vi "Create.vi"(7 "options (all enabled)":T1={"Measure Period"=TRUE, "Measure Rx/Tx Duration"=TRUE}, 8 "error in (no error)":errorcluster) -> (0 "error out":errorcluster, 3 "performance":refnum<class "Performance.lvclass">)   [LabVIEW 2017, in "DSF Core.lvlib" / "Performance.lvclass"]
uses:
  Performance.lvclass
  Typedefs/DSF Performance Options.ctl
  Timing Status/Timing Status Data.ctl
  <vilib>/NI/Memory Manager/Classes/Pointer/Pointer.lvclass/Pointer.ctl
  Performance.lvclass/Performance.ctl
  <vilib>/NI/Memory Manager/Classes/Pointer/Check Size (0D).vi
  <vilib>/NI/Memory Manager/Classes/Pointer/Get Address.vi
  <vilib>/NI/Memory Manager/Classes/Pointer/Check Null Pointer.vi
  Timing Status/Timing Status Size.vi
  <vilib>/NI/Memory Manager/Classes/Pointer/Errors.vi
  <vilib>/NI/Memory Manager/Classes/Pointer/Out of Bounds.vi
  <vilib>/NI/Memory Manager/Classes/Pointer/Get Size.vi
  <vilib>/NI/Memory Manager/Classes/Pointer/Null Pointer.vi
  <vilib>/NI/Memory Manager/Classes/Pointer/Is Null.vi
  <vilib>/NI/Memory Manager/VIs/Source.Write.String.vi
  <vilib>/NI/Memory Manager/Classes/Pointer/Write Pointer Size.vi
  <vilib>/NI/Memory Manager/Classes/Pointer/Create Error.vi
  <vilib>/NI/Memory Manager/VIs/Source.Write.Scalar.Base10.vi
  <vilib>/NI/Memory Manager/VIs/Source.Write.Scalar.Base10 (U64).vi
  <vilib>/NI/Memory Manager/VIs/New Error Cluster Constant.vi
  <vilib>/NI/Memory Manager/VIs/New Error Cluster Constant (512B).vi
  <vilib>/NI/Memory Manager/VIs/Error Cluster.Set Status.vi
  <vilib>/NI/Memory Manager/VIs/Error Cluster.Set Code.vi
  <vilib>/NI/Memory Manager/VIs/Error Cluster.Set VI Source.vi
  <vilib>/NI/Memory Manager/Constants/Constants.vi
  <vilib>/NI/Memory Manager/Constants/Library Name.vi
  <vilib>/NI/Memory Manager/Classes/Pointer/Pointer Error Info.vi
  <vilib>/NI/Memory Manager/Constants/Pointer Class Name.vi
  Timing Status/Timing Status.lvclass
  C:/Program Files (x86)/National Instruments/LabVIEW 2017/vi.lib/NI/Memory Manager/Classes/Pointer/Pointer.lvclass
  DSF Core.lvlib
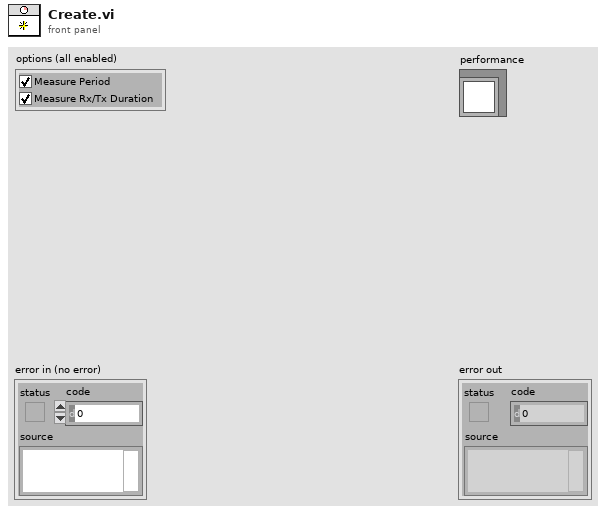
[diagram p1: front panel]
types:
  T1 = typedef "DSF Core.lvlib/DSF Performance Options.ctl" = cluster{"Measure Period":bool, "Measure Rx/Tx Duration":bool}
  T2 = typedef "DSF Core.lvlib/Timing Status.lvclass/Timing Status Data.ctl" = cluster{"rx start time":u32, "rx end time":u32, "tx start time":u32, "tx end time":u32, "cycle start time":u32, "cycle end time":u32, "prev start time":u32}
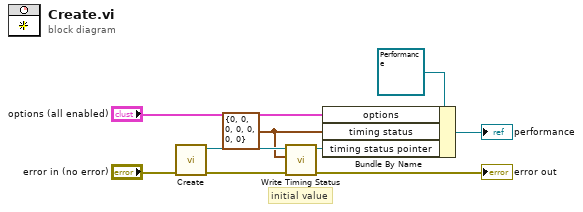
[diagram p0: block diagram]
diagram:
  w3 = T2 {"rx start time"=0, "rx end time"=0, "tx start time"=0, "tx end time"=0, "cycle start time"=0, "cycle end time"=0, "prev start time"=0} ("timing status")
  # "initial value"
  n1 = call "Create.vi"("error in (no error)"="error in (no error)") -> ("error out"=w4:errorcluster, "timing status pointer"=w5:refnum<class "Timing Status.lvclass">)  [unwired: 9 in]
  n2 = call "Write Timing Status.vi"("error in (no error)"=w4, "timing status"=w3, "timing status pointer in"=w5) -> ("error out"=→"error out":errorcluster, "timing status pointer out"=w2:refnum<class "Timing Status.lvclass">)  [unwired: 7 in]
  n3 = Bundle By Name(cluster=refnum<class "Performance.lvclass"> refnum ("Framework Performance in"), "options"="options (all enabled)", "timing status"=w3, "timing status pointer"=w2) -> (→"performance":refnum<class "Performance.lvclass">)
